vi "Load Bitfile.vi"(8 "error in (no error)":errorcluster, 9 "OptionalInfo":T2, 10 "NewVal":path, 11 "Section Ref in":T1 format="%.0x") -> (0 "error out":errorcluster, 2 "version":string, 3 "Section Ref out":T1 format="%.0x")   [LabVIEW 2015, in "Engine Simulation Toolkit System Explorer.lvlib"]
uses:
  Engine Simulation Toolkit System Explorer.lvlib
  <vilib>/NI Veristand/Custom Device API/Dependent File Optional Info.ctl
  <vilib>/NI Veristand/Custom Device API/Custom Device Item Ref.ctl
  Shared/Properties.vi
  <vilib>/NI Veristand/Custom Device API/Set Item Property (Dependent File).vi
  <vilib>/NI Veristand/Custom Device API/Custom Device API.lvlib
  Shared/Engine Simulation Toolkit Shared.lvlib
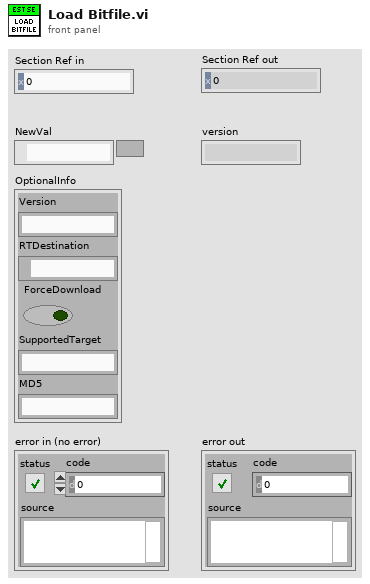
[diagram p1: front panel]
types:
  T1 = typedef "Custom Device API.lvlib/Custom Device Item Ref.ctl" = u64
  T2 = typedef "Custom Device API.lvlib/Dependent File Optional Info.ctl" = cluster{"Version":string, "RTDestination":path, "ForceDownload":bool, "SupportedTarget":string, "MD5":string}
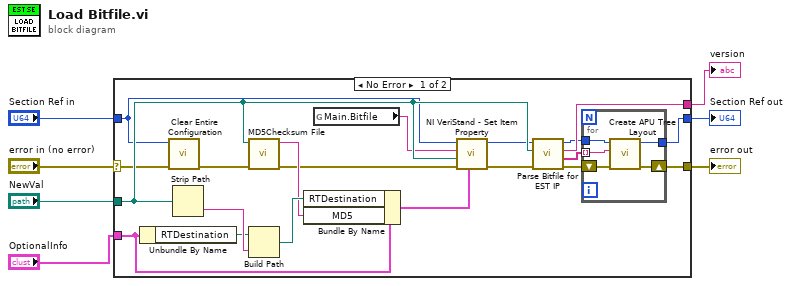
[diagram p0: block diagram]
diagram:
  n1 = case shown="No Error" "error in (no error)" {
    selector: "error in (no error)" -> [w18 w33]
    tunnel: "NewVal" -> [w24 _]
    tunnel: "OptionalInfo" -> [w23 _]
    tunnel: [w22 _] -> w5
    tunnel: "Section Ref in" -> [w20 w34]
    tunnel: [w14 w33] -> w2
    tunnel: [w8 w34] -> w1
    frame No Error {
      n2 = Unbundle By Name(w23) -> ("RTDestination"=w25:path)
      n3 = call "Clear Entire Configuration.vi"("error in (no error)"=w18, "Item Ref in"=w20) -> ("error out"=w19:errorcluster)  [unwired: 9 in]
      n4 = Strip Path(path=w24) -> (name=w27:string)  [unwired: 1 out]
      n5 = call <vilib>:"MD5Checksum File.vi"("error in (no error)"=w19, "Path"=w24) -> ("error out"=w10:errorcluster, "MD5 message-digest"=w11:string)  [unwired: 8 in]
      n6 = Build Path(base path=w25, name or relative path=w27) -> (appended path=w26:path)
      n7 = Bundle By Name(cluster=w23, "RTDestination"=w26, "MD5"=w11) -> (w12:T2)
      n8 = global read "Properties.vi" "Main.Bitfile"() -> (w17:string)
      n9 = call-poly <vilib>:"NI VeriStand - Set Item Property.vi"("OptionalInfo"=w12, "error in (no error)"=w10, "Path"=w24, "Property Name"=w17, "Item Ref in"=w20) -> ("error out"=w9:errorcluster, "Item Ref out"=w13:T1)  [unwired: 4 in, 1 out]
      n10 = call "Parse Bitfile for EST IP.vi"("error in (no error)"=w9, "bitfile path"=w24, "Item Ref in"=w13) -> ("error out"=w21:errorcluster, "APUs"=w16:string[], "version"=w22:string, "Item Ref out"=w15:T1)  [unwired: 5 in]
      n11 = for {
        shift-right: [w31] -> w14
        shift-left: w21 -> [w32]
        tunnel: w15 -> [w30]
        tunnel: w16 -> [w29] mode=indexing
        tunnel: [w28] -> w8
        n12 = call "Create APU Tree Layout.vi"("error in (no error)"=w32, "engine name"=w29, "Section Ptr"=w30) -> ("error out"=w31:errorcluster, "Section Ptr dup"=w28:T1)  [unwired: 6 in, 1 out]
      }
    }
    frame Error {
    }
  }
  "version" <- w5
  "error out" <- w2
  "Section Ref out" <- w1
